vi "ParseReqPDU.vi"(8 "数据in":string) -> (0 "All RY":bool[][](array[boolean]), 1 "All RWw":u16[][](array[numeric]) format="%04x", 2 "从站IP组":u32[](array[numeric]) format="%08x", 3 "主站信息":T2 {"时间戳" format="%016x"; "帧号" format="%04x"; "主站IP" format="%08x"})   [LabVIEW 2018]
panel:
  in  "选项卡控件":T1(tab)
  out "1RX":bool[][](array[boolean]) caption="RY"
  out "1RWr":u16[][](array[numeric]) caption="RWw"
  out "2RX":bool[][](array[boolean]) caption="RY"
  out "2RWr":u16[][](array[numeric]) caption="RWw"
  out "3RX":bool[][](array[boolean]) caption="RY"
  out "3RWr":u16[][](array[numeric]) caption="RWw"
  out "4RX":bool[][](array[boolean]) caption="RY"
  out "4RWr":u16[][](array[numeric]) caption="RWw"
  out "5RX":bool[][](array[boolean]) caption="RY"
  out "5RWr":u16[][](array[numeric]) caption="RWw"
  out "6RX":bool[][](array[boolean]) caption="RY"
  out "6RWr":u16[][](array[numeric]) caption="RWw"
  out "7RX":bool[][](array[boolean]) caption="RY"
  out "7RWr":u16[][](array[numeric]) caption="RWw"
  out "8RX":bool[][](array[boolean]) caption="RY"
  out "8RWr":u16[][](array[numeric]) caption="RWw"
  out "9RX":bool[][](array[boolean]) caption="RY"
  out "9RWr":u16[][](array[numeric]) caption="RWw"
  out "10RX":bool[][](array[boolean]) caption="RY"
  out "10RWr":u16[][](array[numeric]) caption="RWw"
  out "11RX":bool[][](array[boolean]) caption="RY"
  out "11RWr":u16[][](array[numeric]) caption="RWw"
  out "12RX":bool[][](array[boolean]) caption="RY"
  out "12RWr":u16[][](array[numeric]) caption="RWw"
  out "13RX":bool[][](array[boolean]) caption="RY"
  out "13RWr":u16[][](array[numeric]) caption="RWw"
  out "14RX":bool[][](array[boolean]) caption="RY"
  out "14RWr":u16[][](array[numeric]) caption="RWw"
  out "15RX":bool[][](array[boolean]) caption="RY"
  out "15RWr":u16[][](array[numeric]) caption="RWw"
  out "16RX":bool[][](array[boolean]) caption="RY"
  out "16RWr":u16[][](array[numeric]) caption="RWw"
  # "8"
  # "0"
  # "1"
  # "2"
  # "3"
  # "4"
  # "5"
  # "6"
  # "7"
  # "9"
  # "A"
  # "B"
  # "C"
  # "D"
  # "E"
  # "F"
  # "8"
  # "0"
  # "1"
  # "2"
  # "3"
  # "4"
  # "5"
  # "6"
  # "7"
  # "9"
  # "A"
  # "B"
  # "C"
  # "D"
  # "E"
  # "F"
  # "8"
  # "0"
  # "1"
  # "2"
  # "3"
  # "4"
  # "5"
  # "6"
  # "7"
  # "9"
  # "A"
  # "B"
  # "C"
  # "D"
  # "E"
  # "F"
  # "8"
  # "0"
  # "1"
  # "2"
  # "3"
  # "4"
  # "5"
  # "6"
  # "7"
  # "9"
  # "A"
  # "B"
  # "C"
  # "D"
  # "E"
  # "F"
  # "8"
  # "0"
  # "1"
  # "2"
  # "3"
  # "4"
  # "5"
  # "6"
  # "7"
  # "9"
  # "A"
  # "B"
  # "C"
  # "D"
  # "E"
  # "F"
  # "8"
  # "0"
  # "1"
  # "2"
  # "3"
  # "4"
  # "5"
  # "6"
  # "7"
  # "9"
  # "A"
  # "B"
  # "C"
  # "D"
  # "E"
  # "F"
  # "8"
  # "0"
  # "1"
  # "2"
  # "3"
  # "4"
  # "5"
  # "6"
  # "7"
  # "9"
  # "A"
  # "B"
  # "C"
  # "D"
  # "E"
  # "F"
  # "8"
  # "0"
  # "1"
  # "2"
  # "3"
  # "4"
  # "5"
  # "6"
  # "7"
  # "9"
  # "A"
  # "B"
  # "C"
  # "D"
  # "E"
  # "F"
  # "8"
  # "0"
  # "1"
  # "2"
  # "3"
  # "4"
  # "5"
  # "6"
  # "7"
  # "9"
  # "A"
  # "B"
  # "C"
  # "D"
  # "E"
  # "F"
  # "8"
  # "0"
  # "1"
  # "2"
  # "3"
  # "4"
  # "5"
  # "6"
  # "7"
  # "9"
  # "A"
  # "B"
  # "C"
  # "D"
  # "E"
  # "F"
  # "8"
  # "0"
  # "1"
  # "2"
  # "3"
  # "4"
  # "5"
  # "6"
  # "7"
  # "9"
  # "A"
  # "B"
  # "C"
  # "D"
  # "E"
  # "F"
  # "8"
  # "0"
  # "1"
  # "2"
  # "3"
  # "4"
  # "5"
  # "6"
  # "7"
  # "9"
  # "A"
  # "B"
  # "C"
  # "D"
  # "E"
  # "F"
  # "8"
  # "0"
  # "1"
  # "2"
  # "3"
  # "4"
  # "5"
  # "6"
  # "7"
  # "9"
  # "A"
  # "B"
  # "C"
  # "D"
  # "E"
  # "F"
  # "8"
  # "0"
  # "1"
  # "2"
  # "3"
  # "4"
  # "5"
  # "6"
  # "7"
  # "9"
  # "A"
  # "B"
  # "C"
  # "D"
  # "E"
  # "F"
  # "8"
  # "0"
  # "1"
  # "2"
  # "3"
  # "4"
  # "5"
  # "6"
  # "7"
  # "9"
  # "A"
  # "B"
  # "C"
  # "D"
  # "E"
  # "F"
  # "8"
  # "0"
  # "1"
  # "2"
  # "3"
  # "4"
  # "5"
  # "6"
  # "7"
  # "9"
  # "A"
  # "B"
  # "C"
  # "D"
  # "E"
  # "F"
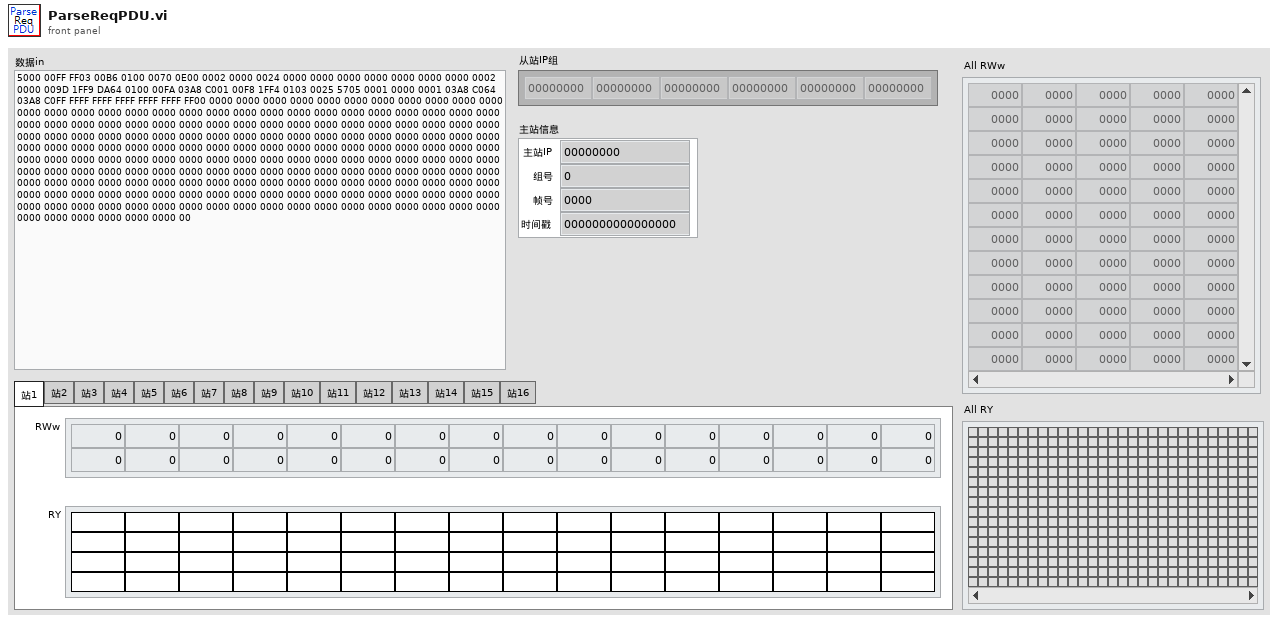
[diagram p1: front panel]
types:
  T1 = enum32{"站1", "站2", "站3", "站4", "站5", "站6", "站7", "站8", "站9", "站10", "站11", "站12", "站13", "站14", "站15", "站16"}
  T2 = cluster{"主站IP":u32, "组号":u8, "帧号":u16, "时间戳":u64}
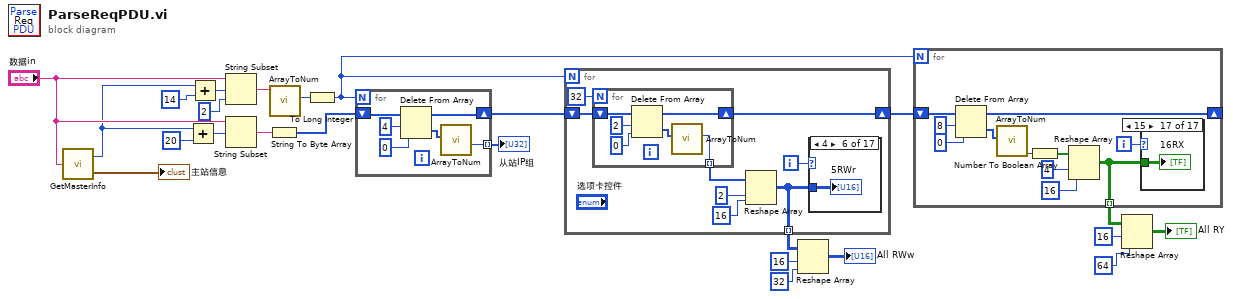
[diagram p0: block diagram]
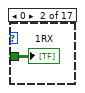
[diagram p3: hidden frame]
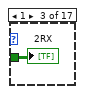
[diagram p4: hidden frame]
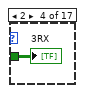
[diagram p5: hidden frame]
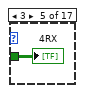
[diagram p6: hidden frame]
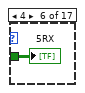
[diagram p7: hidden frame]
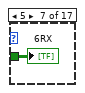
[diagram p8: hidden frame]
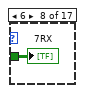
[diagram p9: hidden frame]
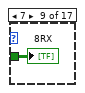
[diagram p10: hidden frame]
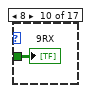
[diagram p11: hidden frame]
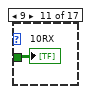
[diagram p12: hidden frame]
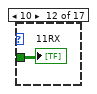
[diagram p13: hidden frame]
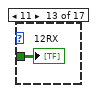
[diagram p14: hidden frame]
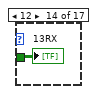
[diagram p15: hidden frame]
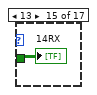
[diagram p16: hidden frame]
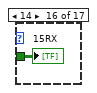
[diagram p17: hidden frame]
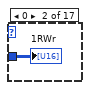
[diagram p19: hidden frame]
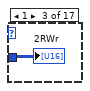
[diagram p20: hidden frame]
diagram:
  n1 = call "GetMasterInfo.vi"("数据in"="数据in") -> ("主站信息"=→"主站信息":T2, "cyclicInfo"=w2:i32)  [unwired: 3 in]
  n2 = Add(x=w2, y=20 ("索引")) -> (x+y=w4:i32)
  n3 = Add(x=w2, y=14 ("索引")) -> (x+y=w5:i32)
  n4 = String Subset ("截取字符串")(string="数据in", offset (0)=w5, length (rest)=2 ("长度")) -> (substring=w24:string)
  n5 = String Subset(string="数据in", offset (0)=w4) -> (substring=w9:string)  [unwired: 1 in]
  n6 = String To Byte Array(string=w9) -> (unsigned byte array=w8:u8[])
  n7 = call "ArrayToNum.vi"("输入字符串"=w24) -> ("2B"=w23:u16)  [unwired: 3 in, 3 out]
  n8 = To Long Integer(number=w23) -> (32bit integer=w19:i32)
  n9 = for {
    N: w19 -> [_]
    shift-right: [w28] -> w21
    shift-left: w8 -> [w30]
    tunnel: [w27] -> w22 mode=indexing
    n10 = Delete From Array(array=w30, length=4 ("长度"), index=0 ("索引")) -> (deleted portion=w25:u8[], array with subset deleted=w28:u8[])
    n11 = call "ArrayToNum.vi"("输入数组"=w25) -> ("4B"=w27:u32)  [unwired: 3 in, 3 out]
  }
  "从站IP组" <- w22
  n12 = for {
    N: w19 -> [_]
    shift-right: [w36] -> w20
    shift-left: w21 -> [w38]
    tunnel: [w32] -> w18 mode=indexing
    i -> [w33]
    n13 = for {
      N: 32 -> [_]
      shift-right: [w57] -> w36
      shift-left: w38 -> [w60]
      tunnel: [w56] -> w31 mode=indexing
      n14 = Delete From Array(array=w60, length=2 ("长度"), index=0 ("索引")) -> (deleted portion=w55:u8[], array with subset deleted=w57:u8[])
      n15 = call "ArrayToNum.vi"("输入数组"=w55) -> ("2B"=w56:u16)  [unwired: 3 in, 3 out]
    }
    n16 = Reshape Array(w31, 2 ("维数大小"), 16 ("维数大小")) -> (w32:u16[][])
    n17 = case shown="4" w33 {
      tunnel: w32 -> [_ w39 w40 w41 w42 w43 w44 w45 w46 w47 w48 w49 w50 w51 w52 w53 w54]
      frame -1, Default {
      }
      frame 0 {
        "1RWr" <- w39
      }
      frame 1 {
        "2RWr" <- w40
      }
      frame 2 {
        "3RWr" <- w41
      }
      frame 3 {
        "4RWr" <- w42
      }
      frame 4 {
        "5RWr" <- w43
      }
      frame 5 {
        "6RWr" <- w44
      }
      frame 6 {
        "7RWr" <- w45
      }
      frame 7 {
        "8RWr" <- w46
      }
      frame 8 {
        "9RWr" <- w47
      }
      frame 9 {
        "10RWr" <- w48
      }
      frame 10 {
        "11RWr" <- w49
      }
      frame 11 {
        "12RWr" <- w50
      }
      frame 12 {
        "13RWr" <- w51
      }
      frame 13 {
        "14RWr" <- w52
      }
      frame 14 {
        "15RWr" <- w53
      }
      frame 15 {
        "16RWr" <- w54
      }
    }
  }
  n18 = Reshape Array(w18, 16 ("维数大小"), 32 ("维数大小")) -> (→"All RWw":u16[][])
  n19 = for {
    N: w19 -> [_]
    shift-right: [w68] -> _
    shift-left: w20 -> [w71]
    tunnel: [w62] -> w13 mode=indexing
    i -> [w66]
    n20 = Delete From Array(array=w71, length=8 ("长度"), index=0 ("索引")) -> (deleted portion=w61:u8[], array with subset deleted=w68:u8[])
    n21 = call "ArrayToNum.vi"("输入数组"=w61) -> ("8B"=w67:u64)  [unwired: 3 in, 3 out]
    n22 = Number To Boolean Array(number=w67) -> (Boolean array=w65:bool[])
    n23 = Reshape Array(w65, 4 ("维数大小"), 16 ("维数大小")) -> (w62:bool[][])
    n24 = case shown="15" w66 {
      tunnel: w62 -> [_ w72 w73 w74 w75 w76 w77 w78 w79 w80 w81 w82 w83 w84 w85 w86 w87]
      frame -1, Default {
      }
      frame 0 {
        "1RX" <- w72
      }
      frame 1 {
        "2RX" <- w73
      }
      frame 2 {
        "3RX" <- w74
      }
      frame 3 {
        "4RX" <- w75
      }
      frame 4 {
        "5RX" <- w76
      }
      frame 5 {
        "6RX" <- w77
      }
      frame 6 {
        "7RX" <- w78
      }
      frame 7 {
        "8RX" <- w79
      }
      frame 8 {
        "9RX" <- w80
      }
      frame 9 {
        "10RX" <- w81
      }
      frame 10 {
        "11RX" <- w82
      }
      frame 11 {
        "12RX" <- w83
      }
      frame 12 {
        "13RX" <- w84
      }
      frame 13 {
        "14RX" <- w85
      }
      frame 14 {
        "15RX" <- w86
      }
      frame 15 {
        "16RX" <- w87
      }
    }
  }
  n25 = Reshape Array(w13, 16 ("维数大小"), 64 ("维数大小")) -> (→"All RY":bool[][])
